vi "Split Divided Segment.vi"(8 "error in (no error)":errorcluster, 9 "tf Modified? in":bool, 10 "Wfm Segment in":T1, 11 "Waveform Buffer in":refnum<class "Waveform Buffer.lvclass">) -> (0 "error out":errorcluster, 1 "tf Modified? out":bool[](array[boolean]), 2 "Segments out":T1[](array[typedef]), 3 "Waveform Buffer out":refnum<class "Waveform Buffer.lvclass">)   [LabVIEW 2015, in "Waveform Buffer.lvclass"]
uses:
  Waveform Buffer.lvclass
  Wfm Segment.ctl
  Data Point.ctl
  Waveform Buffer.lvclass/Waveform Buffer.ctl
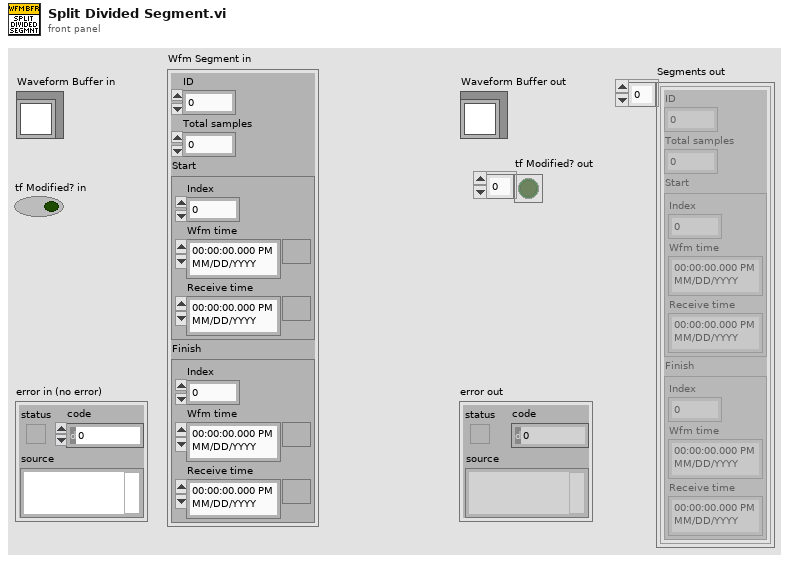
[diagram p1: front panel]
types:
  T1 = typedef "Waveform Buffer.lvclass/Wfm Segment.ctl" = cluster{"ID":u64, "Total samples":i32, "Start":T2, "Finish":T2}
  T2 = typedef "Waveform Buffer.lvclass/Data Point.ctl" = cluster{"Index":i32, "Wfm time":timestamp, "Receive time":timestamp}
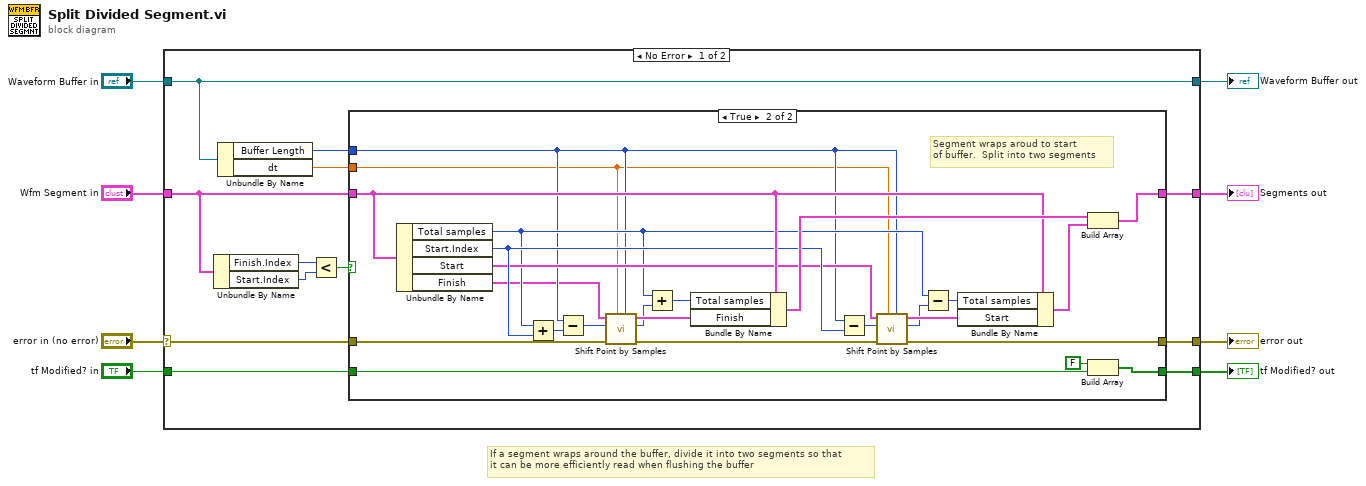
[diagram p0: block diagram]
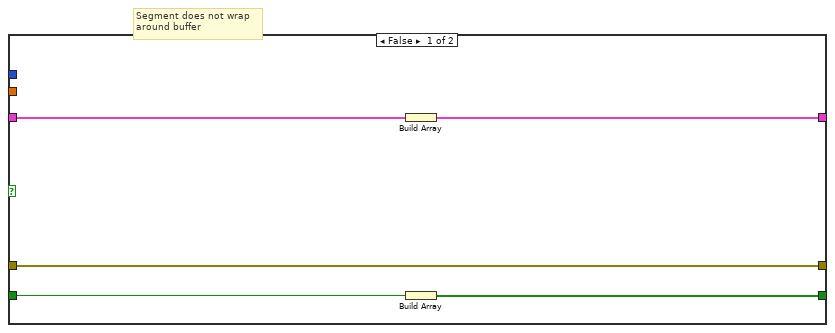
[diagram p2: hidden frame]
diagram:
  # "If a segment wraps around the buffer, divide it into two segments so that\nit can be more efficiently read when flushing the buffer"
  n1 = case shown="No Error" "error in (no error)" {
    selector: "error in (no error)" -> [w11 w52]
    tunnel: [w12 w52] -> w7
    tunnel: [w15 w51] -> w5
    tunnel: "Waveform Buffer in" -> [w15 w51]
    tunnel: "Wfm Segment in" -> [w17 _]
    tunnel: [w16 _] -> w3
    tunnel: "tf Modified? in" -> [w10 _]
    tunnel: [w9 _] -> w1
    frame No Error {
      n2 = Unbundle By Name(w17) -> ("Finish.Index"=w20:i32, "Start.Index"=w19:i32)
      n3 = Unbundle By Name(w15) -> ("Buffer Length"=w14:i32, "dt"=w13:dbl)
      n4 = Less?(x=w20, y=w19) -> (x < y?=w18:bool)
      n5 = case shown="True" w18 {
        tunnel: w17 -> [w25 w47]
        tunnel: [w24 w48] -> w16
        tunnel: w14 -> [_ w31]
        tunnel: w13 -> [_ w30]
        tunnel: [w23 w33] -> w12
        tunnel: w11 -> [w23 w32]
        tunnel: w10 -> [w22 w28]
        tunnel: [w21 w26] -> w9
        frame False {
          # "Segment does not wrap\naround buffer"
          n6 = Build Array(w25) -> (w24:T1[])
          n7 = Build Array(w22) -> (w21:bool[])
        }
        frame True {
          # "Segment wraps aroud to start\nof buffer.  Split into two segments"
          n8 = Unbundle By Name(w47) -> ("Total samples"=w36:i32, "Start.Index"=w42:i32, "Start"=w40:T2, "Finish"=w29:T2)
          n9 = Add(x=w36, y=w42) -> (x+y=w44:i32)
          n10 = Subtract(x=w31, y=w44) -> (x-y=w43:i32)
          n11 = call "Shift Point by Samples.vi"("Buffer Length"=w31, "dt"=w30, "error in (no error)"=w32, "Samples"=w43, "Data Point in"=w29) -> ("error out"=w34:errorcluster, "Samples dup"=w38:i32, "Data Point out"=w46:T2)  [unwired: 4 in]
          n12 = Add(x=w36, y=w38) -> (x+y=w39:i32)
          n13 = Bundle By Name(cluster=w47, "Total samples"=w39, "Finish"=w46) -> (w50:T1)
          n14 = Subtract(x=w31, y=w42) -> (x-y=w41:i32)
          n15 = call "Shift Point by Samples.vi"("Buffer Length"=w31, "dt"=w30, "error in (no error)"=w34, "Samples"=w41, "Data Point in"=w40) -> ("error out"=w33:errorcluster, "Samples dup"=w35:i32, "Data Point out"=w45:T2)  [unwired: 4 in]
          n16 = Subtract(x=w36, y=w35) -> (x-y=w37:i32)
          n17 = Bundle By Name(cluster=w47, "Total samples"=w37, "Start"=w45) -> (w49:T1)
          n18 = Build Array(w50, w49) -> (w48:T1[])
          n19 = Build Array(FALSE, w28) -> (w26:bool[])
        }
      }
    }
    frame Error {
    }
  }
  "error out" <- w7
  "Waveform Buffer out" <- w5
  "Segments out" <- w3
  "tf Modified? out" <- w1
